vi "Read Frame Data.vi"(8 "error in":errorcluster, 11 "XNET Frames":refnum<k21>[](array[refnum])) -> (0 "error out":errorcluster, 3 "Frames":T1[](array[typedef]))   [LabVIEW 2020, in "Communication Bus Template System Explorer.lvlib" / "Implementation.lvlib"]
uses:
  Types/Frame.ctl
  Types/Signal.ctl
  Implementation.lvlib
  <resource>/objmgr/xnet.rc
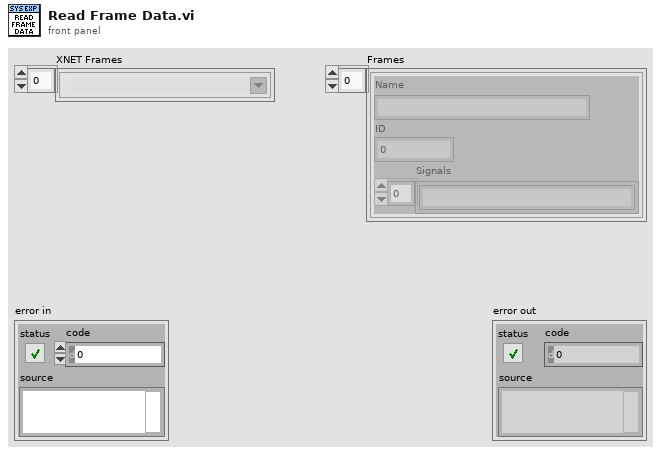
[diagram p1: front panel]
types:
  T1 = typedef "Communication Bus Template System Explorer.lvlib/Implementation.lvlib/Frame.ctl" = cluster{"Name":string, "ID":u32, "Signals":T2[]}
  T2 = typedef "Communication Bus Template System Explorer.lvlib/Implementation.lvlib/Signal.ctl" = string
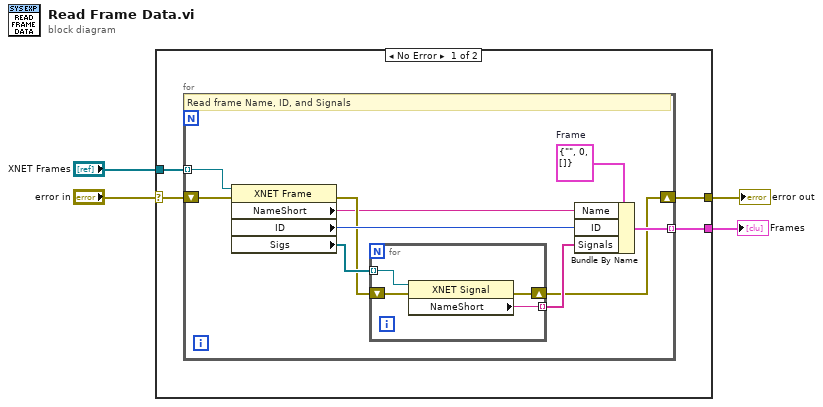
[diagram p0: block diagram]
diagram:
  n1 = case shown="No Error" "error in" {
    selector: "error in" -> [w5 w23]
    tunnel: [w8 _] -> w4
    tunnel: "XNET Frames" -> [w7 _]
    tunnel: [w6 w23] -> w2
    frame No Error {
      n2 = for {
        tunnel: w7 -> [w18] mode=indexing
        tunnel: [w14] -> w8 mode=indexing
        shift-right: [w12] -> w6
        shift-left: w5 -> [w13]
        w9 = T1 {"Name"="", "ID"=0, "Signals"=[]}  # Frame
        # "Read frame Name, ID, and Signals"
        n3 = property class="XNET Frame"(reference=w18, error in=w13) -> (error out=w11:errorcluster, "NameShort"=w10:string, "ID"=w16:u32, "Sigs"=w17:refnum<k21>[])  [unwired: 1 out]
        n4 = for {
          tunnel: w17 -> [w22] mode=indexing
          tunnel: [w21] -> w15 mode=indexing
          shift-right: [w19] -> w12
          shift-left: w11 -> [w20]
          n5 = property class="XNET Signal"(reference=w22, error in=w20) -> (error out=w19:errorcluster, "NameShort"=w21:string)  [unwired: 1 out]
        }
        n6 = Bundle By Name(cluster=w9, "Name"=w10, "ID"=w16, "Signals"=w15) -> (w14:T1)
      }
    }
    frame Error {
    }
  }
  "Frames" <- w4
  "error out" <- w2
